vi "getLinesForVolume.vi"(10 "volume num":u32, 11 "Array of lines":T1[](array[typedef])) -> (0 "out of lines":bool, 1 "lines lost":i32, 2 "lines for current volume":T1[](array[typedef]), 3 "lines for future volume":T1[](array[typedef]))   [LabVIEW 2010]
uses:
  line_info.ctl
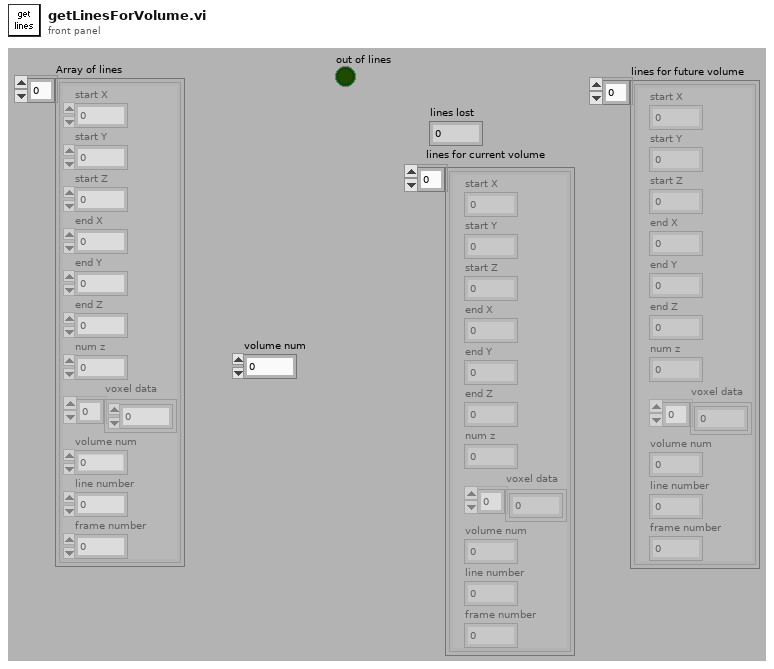
[diagram p1: front panel]
types:
  T1 = typedef "line_info.ctl" = cluster{"start X":i16, "start Y":i16, "start Z":i16, "end X":i16, "end Y":i16, "end Z":i16, "num z":u8, "voxel data":u32[], "volume num":u32, "line number":u16, "frame number":u16}
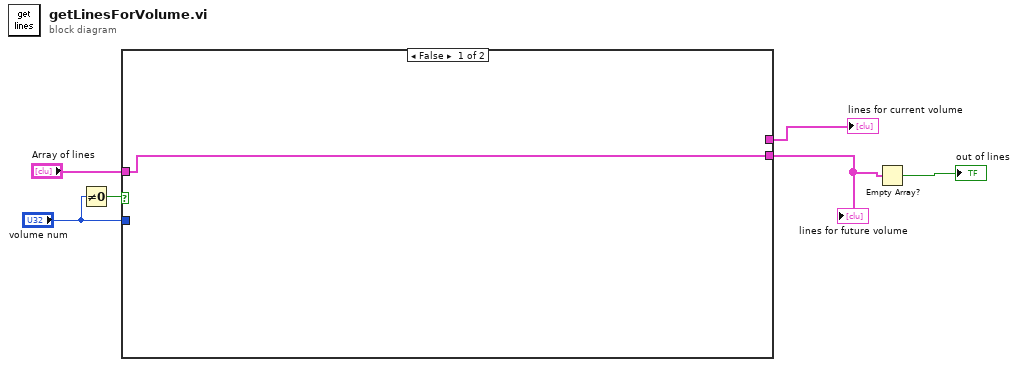
[diagram p0: block diagram]
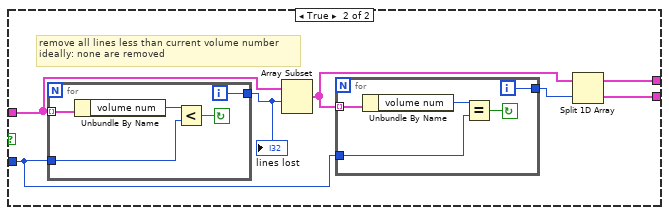
[diagram p2: hidden frame]
diagram:
  n1 = Not Equal To 0?(x="volume num") -> (x != 0?=w2:bool)
  n2 = case shown="False" w2 {
    tunnel: "Array of lines" -> [w7 w14]
    tunnel: "volume num" -> [_ w12]
    tunnel: [_ w9] -> w5
    tunnel: [w7 w8] -> w4
    frame False {
    }
    frame True {
      # "remove all lines less than current volume number\nideally: none are removed"
      n3 = for {
        tunnel: w14 -> [w24] mode=indexing
        tunnel: w12 -> [w22]
        tunnel: [w20] -> w13
        i -> [w20]
        stop <- w21 continue-if-true
        n4 = Unbundle By Name(w24) -> ("volume num"=w23:u32)
        n5 = Less?(x=w23, y=w22) -> (x < y?=w21:bool)
      }
      "lines lost" <- w13
      n6 = Array Subset(array=w14, index=w13) -> (w11:T1[])  [unwired: 1 in]
      n7 = for {
        tunnel: w11 -> [w19] mode=indexing
        tunnel: w12 -> [w17]
        tunnel: [w15] -> w10
        i -> [w15]
        stop <- w16 continue-if-true
        n8 = Unbundle By Name(w19) -> ("volume num"=w18:u32)
        n9 = Equal?(x=w18, y=w17) -> (x = y?=w16:bool)
      }
      n10 = Split 1D Array(array=w11, index=w10) -> (first subarray=w9:T1[], second subarray=w8:T1[])
    }
  }
  "lines for current volume" <- w5
  "lines for future volume" <- w4
  n11 = Empty Array?(array=w4) -> (empty?=→"out of lines":bool)
